vi "closePanel.vi"() -> ()   [LabVIEW 2015]
uses:
  GlobalPath.vi
  GlobalData.vi
  GlobalVi.vi
panel:
  out "Debug":string=" PANEL CLOSURE:"
  out "Stiffback XY Filename":string
  out "Micrometer Diff Filename":string
  out "PanelName":string
  in  "Done with gauge system?":bool
  in  "Done with micrometer?":bool
  in  "Open micrometer dry run":bool
  in  "Open Stiffback XY Program":bool
  in  "DONE ALL?":bool
  in  "ptfe 12":bool caption="Wait 24h for the glue to cure"
  in  "ptfe 11":bool caption="Remove the movement arch from over the table"
  in  "ptfe 8":bool caption="Position the weights on the stiffback"
  in  "ptfe 7":bool caption="Release the stiffback from the movement arch"
  in  "ptfe 6":bool caption="Lower the stiffback on the reference plates"
  in  "ptfe 5":bool caption="Move the stiffback over the reference plates"
  in  "ptfe 4":bool caption="Rotate the stiffback upside down"
  in  "ptfe 3":bool caption="Check cleanness of the 20 stiffback supports"
  in  "ptfe 2":bool caption="Move the stiffback away from the table"
  # "1. Panel Closure"
  # "2. Measurements"
  # "Micrometer measurement of the distance between the reference plates \nand the stiffback plates along the perimeter"
  # "Stiffback surface measurement (back side) with \ngauge system"
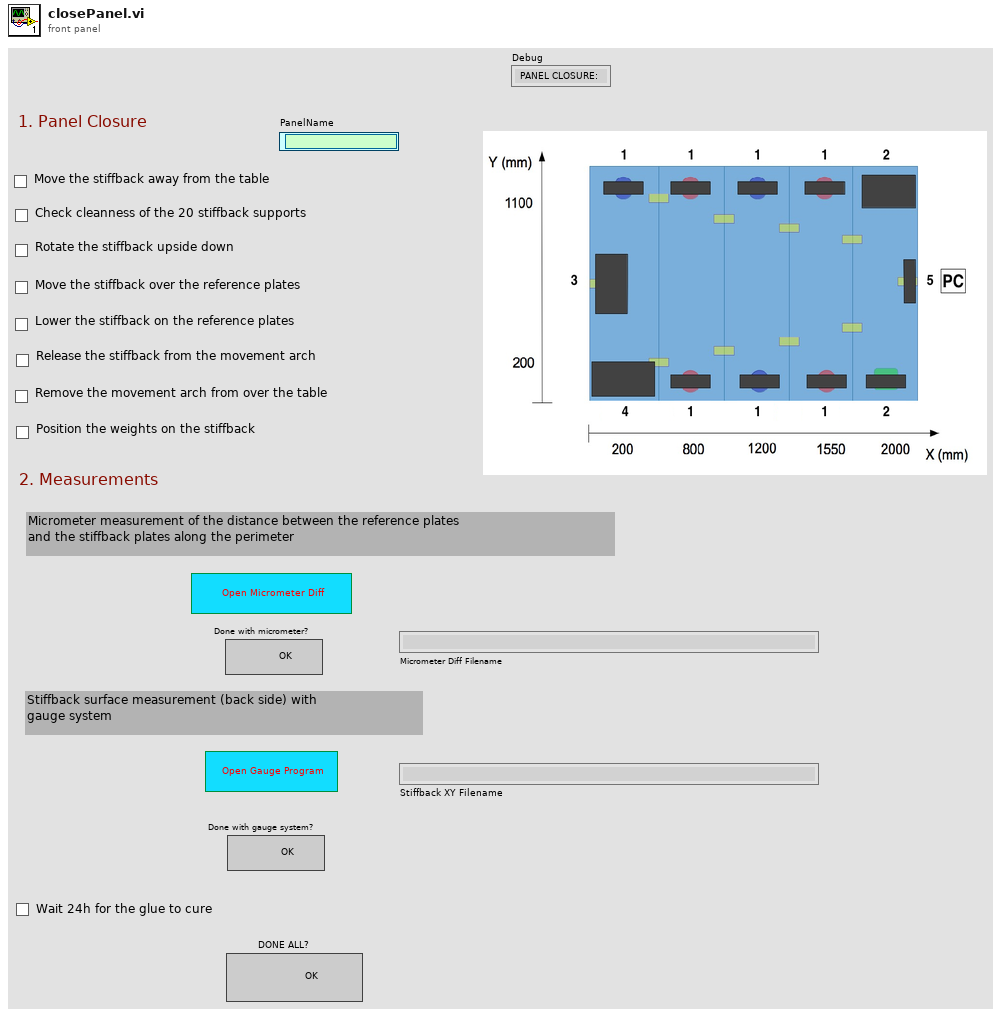
[diagram p1: front panel]
types:
  T1 = enum16{"open", "replace", "create", "open or create", "replace or create", "replace or create with confirmation"}
  T2 = enum32{"Bad", "Idle", "Run top level", "Running"}
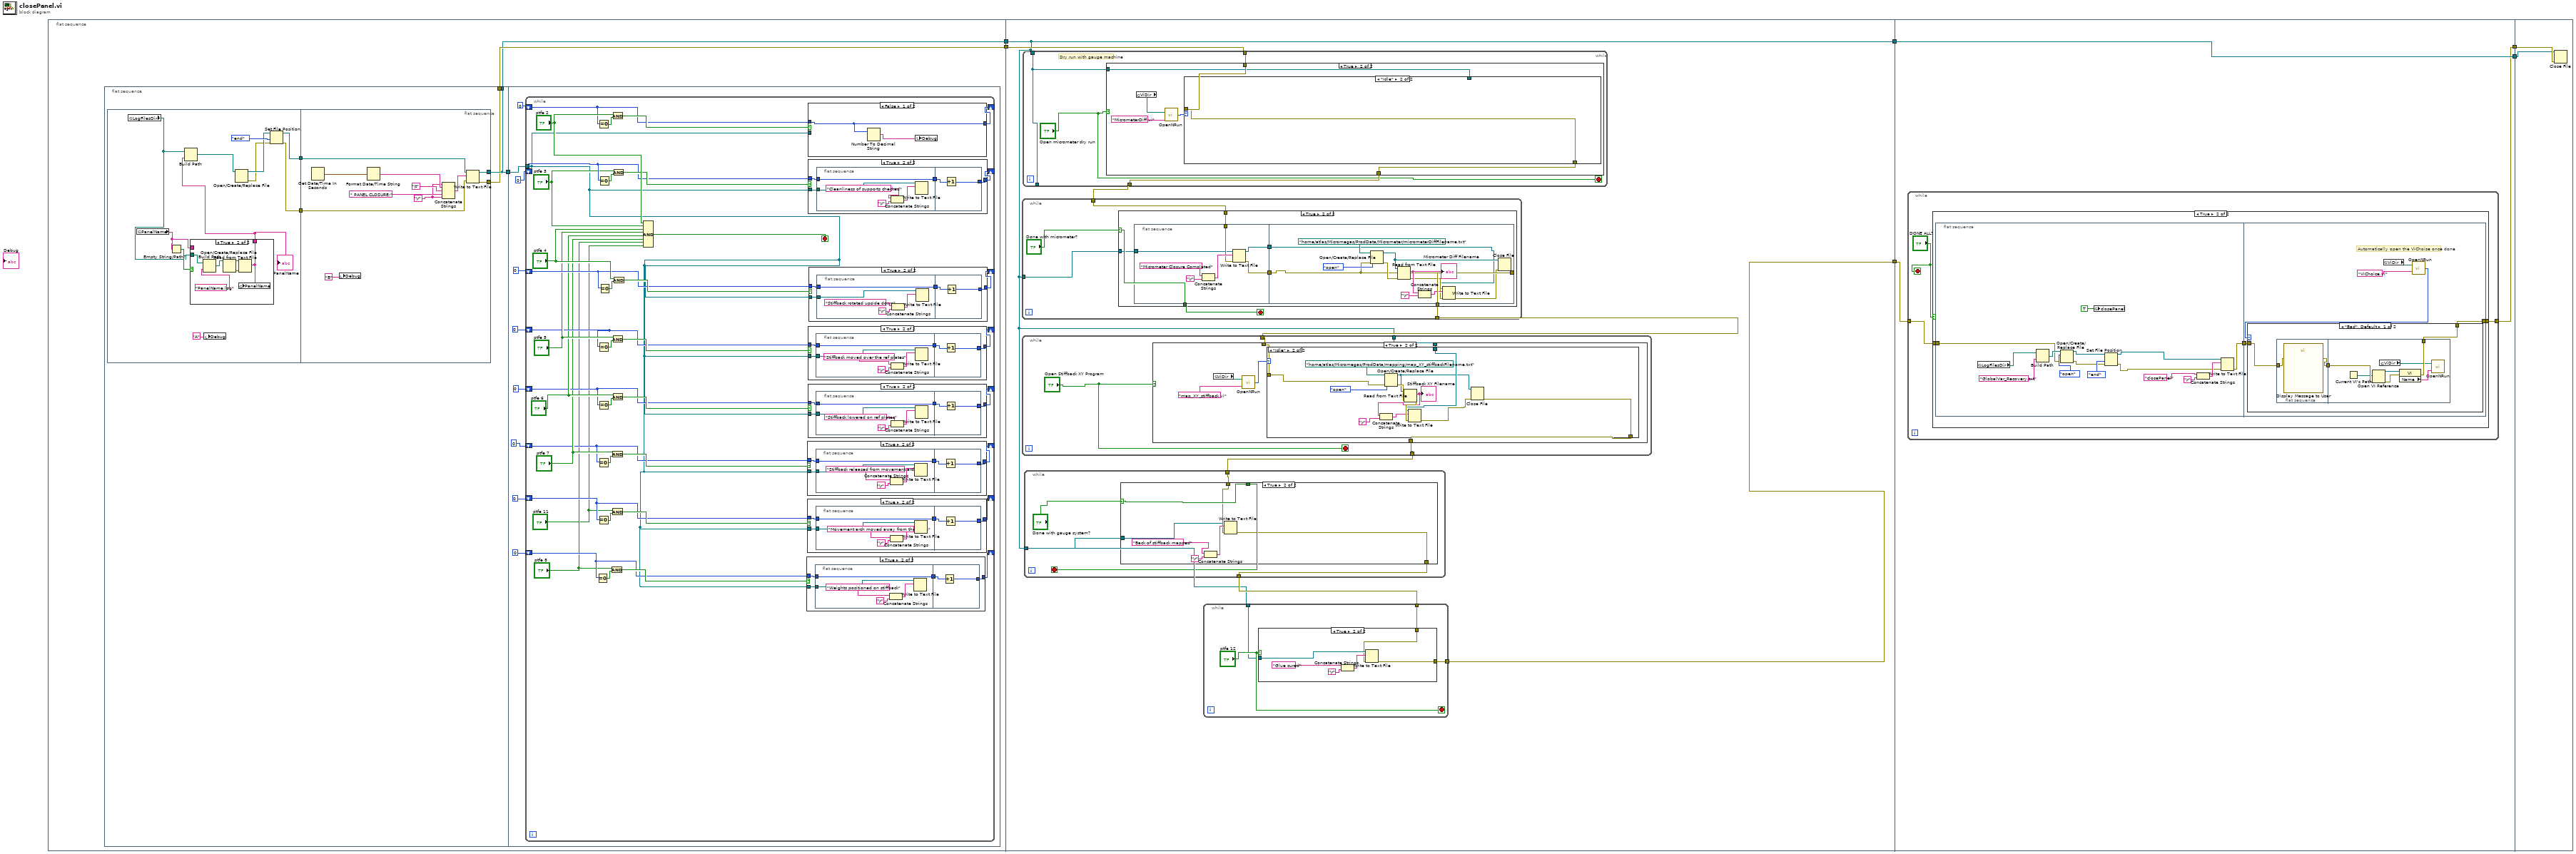
[diagram p0: block diagram]
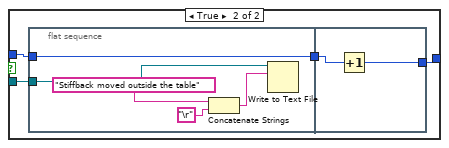
[diagram p10: hidden frame]
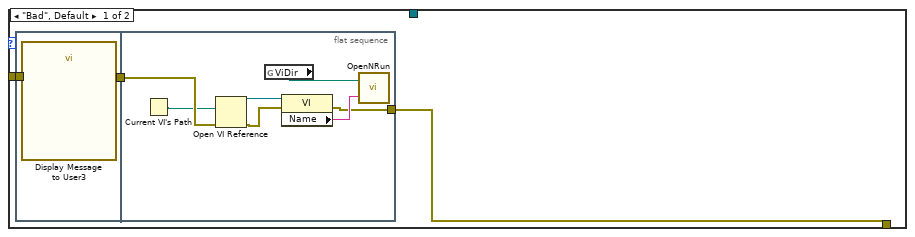
[diagram p14: hidden frame]
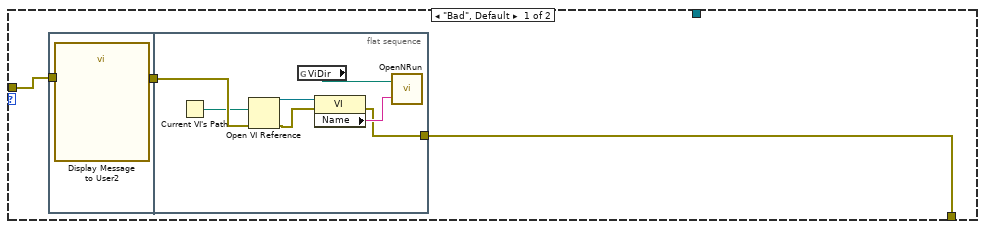
[diagram p16: hidden frame]
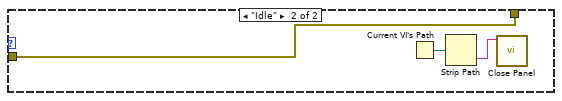
[diagram p19: hidden frame]
diagram:
  n1 = flat-sequence {
    tunnel: [w8] -> w4
    tunnel: [w7] -> w2
    tunnel: w4 -> [w197]
    tunnel: [w192] -> w3
    tunnel: w2 -> [w191]
    tunnel: [w191] -> w1
    tunnel: [w313] -> w6
    tunnel: w3 -> [w314]
    tunnel: w1 -> [w315]
    tunnel: [w315] -> w5
    tunnel: w6 -> [w359]
    tunnel: w5 -> [w358]
    frame #0 {
      n2 = flat-sequence {
        tunnel: [w12] -> w9
        tunnel: [w12] -> w7
        tunnel: [w11] -> w8
        tunnel: w9 -> [w51]
        frame #0 {
          n3 = flat-sequence {
            tunnel: [w22] -> w13
            tunnel: [w19] -> w10
            tunnel: w13 -> [w39]
            tunnel: [w38] -> w12
            tunnel: [w37] -> w11
            tunnel: w10 -> [w36]
            frame #0 {
              n4 = global read "GlobalPath.vi" "LogFilesDir"() -> (w15:path)
              n5 = global read "GlobalData.vi" "PanelName"() -> (w18:string)
              n6 = Empty String/Path?(string/path=w18) -> (empty?=w17:bool)
              n7 = case shown="True" w17 {
                tunnel: w15 -> [_ w31]
                tunnel: [w25 w26] -> w16
                tunnel: w18 -> [w25 _]
                frame False {
                }
                frame True {
                  n8 = Build Path(base path=w31, name or relative path="PanelName.log") -> (appended path=w30:path)
                  n9 = Open/Create/Replace File(file path (use dialog)=w30) -> (refnum out=w27:refnum<file>, error out=w28:errorcluster)  [unwired: 5 in, 1 out]
                  n10 = Read from Text File(file (use dialog)=w27, error in=w28) -> (text=w26:string)  [unwired: 2 in, 3 out]
                  n11 = global write "GlobalData.vi" "PanelName"(w26) -> ()
                }
              }
              "PanelName" <- w16
              n12 = Build Path(base path=w15, name or relative path=w16) -> (appended path=w24:path)
              n13 = local write "Debug"("A") -> ()
              n14 = Open/Create/Replace File(file path (use dialog)=w24) -> (refnum out=w21:refnum<file>, error out=w20:errorcluster)  [unwired: 5 in, 1 out]
              n15 = Set File Position(refnum=w21, from (0:start)=enum16{"start", "end", "current"}."end", error in=w20) -> (refnum out=w22:refnum<file>, error out=w19:errorcluster)  [unwired: 1 in]
            }
            frame #1 {
              w33 = "\r"
              n16 = Get Date/Time In Seconds() -> (seconds since 1Jan1904=w35:timestamp)
              n17 = local write "Debug"("B") -> ()
              n18 = Format Date/Time String(seconds (now)=w35) -> (date/time string=w41:string)  [unwired: 2 in]
              n19 = Concatenate Strings(w33, w41, "\t", " PANEL CLOSURE:", w33) -> (w40:string)
              n20 = Write to Text File(file (use dialog)=w39, text=w40, error in=w36) -> (refnum out=w38:refnum<file>, error out=w37:errorcluster)  [unwired: 1 in, 1 out]
            }
          }
        }
        frame #1 {
          n21 = while {
            tunnel: w51 -> [w53]
            shift-right: [w89] -> _
            shift-left: 0 -> [w52]
            shift-right: [w85] -> _
            shift-left: 0 -> [w86]
            shift-right: [w79] -> _
            shift-left: 0 -> [w80]
            shift-right: [w74] -> _
            shift-left: 0 -> [w75]
            shift-right: [w69] -> _
            shift-left: 0 -> [w70]
            shift-right: [w64] -> _
            shift-left: 0 -> [w65]
            shift-right: [w56] -> _
            shift-left: 0 -> [w59]
            shift-right: [w55] -> _
            shift-left: 0 -> [w58]
            stop <- w93 stop-if-true
            n22 = Equal To 0?(x=w58) -> (x = 0?=w61:bool)
            n23 = Equal To 0?(x=w65) -> (x = 0?=w68:bool)
            n24 = Equal To 0?(x=w59) -> (x = 0?=w63:bool)
            n25 = Equal To 0?(x=w52) -> (x = 0?=w92:bool)
            n26 = Equal To 0?(x=w75) -> (x = 0?=w78:bool)
            n27 = Equal To 0?(x=w70) -> (x = 0?=w73:bool)
            n28 = Equal To 0?(x=w86) -> (x = 0?=w88:bool)
            n29 = Equal To 0?(x=w80) -> (x = 0?=w83:bool)
            n30 = And(x="ptfe 8", y=w61) -> (x .and. y?=w60:bool)
            n31 = And(x="ptfe 7", y=w68) -> (x .and. y?=w67:bool)
            n32 = And(x="ptfe 11", y=w63) -> (x .and. y?=w62:bool)
            n33 = And(x="ptfe 2", y=w92) -> (x .and. y?=w91:bool)
            n34 = And(x="ptfe 5", y=w78) -> (x .and. y?=w77:bool)
            n35 = And(x="ptfe 6", y=w73) -> (x .and. y?=w72:bool)
            n36 = And(x="ptfe 3", y=w88) -> (x .and. y?=w87:bool)
            n37 = And(x="ptfe 4", y=w83) -> (x .and. y?=w82:bool)
            n38 = Compound Arithmetic op=AND("ptfe 2", "ptfe 3", "ptfe 4", "ptfe 5", "ptfe 6", "ptfe 7", "ptfe 8", "ptfe 11") -> (w93:bool)
            n39 = case shown="True" w60 {
              tunnel: w53 -> [_ w98]
              tunnel: w58 -> [w94 w96]
              tunnel: [w94 w95] -> w55
              frame False {
              }
              frame True {
                n40 = flat-sequence {
                  tunnel: w98 -> [w101]
                  tunnel: [w100] -> w97
                  tunnel: w96 -> [w100]
                  tunnel: w97 -> [w105]
                  tunnel: [w104] -> w95
                  frame #0 {
                    n41 = Concatenate Strings("Weights positioned on stiffback", "\r") -> (w103:string)
                    n42 = Write to Text File(file (use dialog)=w101, text=w103) -> ()  [unwired: 2 in, 3 out]
                  }
                  frame #1 {
                    n43 = Increment(x=w105) -> (x+1=w104:i32)
                  }
                }
              }
            }
            n44 = case shown="True" w67 {
              tunnel: w53 -> [_ w122]
              tunnel: w65 -> [w118 w120]
              tunnel: [w118 w119] -> w64
              frame False {
              }
              frame True {
                n45 = flat-sequence {
                  tunnel: w122 -> [w125]
                  tunnel: [w124] -> w121
                  tunnel: w120 -> [w124]
                  tunnel: w121 -> [w129]
                  tunnel: [w128] -> w119
                  frame #0 {
                    n46 = Concatenate Strings("Stiffback released from movement arch", "\r") -> (w127:string)
                    n47 = Write to Text File(file (use dialog)=w125, text=w127) -> ()  [unwired: 2 in, 3 out]
                  }
                  frame #1 {
                    n48 = Increment(x=w129) -> (x+1=w128:i32)
                  }
                }
              }
            }
            n49 = case shown="True" w62 {
              tunnel: w53 -> [_ w110]
              tunnel: w59 -> [w106 w108]
              tunnel: [w106 w107] -> w56
              frame False {
              }
              frame True {
                n50 = flat-sequence {
                  tunnel: w110 -> [w113]
                  tunnel: [w112] -> w109
                  tunnel: w108 -> [w112]
                  tunnel: w109 -> [w117]
                  tunnel: [w116] -> w107
                  frame #0 {
                    n51 = Concatenate Strings("Movement arch moved away from the table", "\r") -> (w115:string)
                    n52 = Write to Text File(file (use dialog)=w113, text=w115) -> ()  [unwired: 2 in, 3 out]
                  }
                  frame #1 {
                    n53 = Increment(x=w117) -> (x+1=w116:i32)
                  }
                }
              }
            }
            n54 = case shown="False" w91 {
              tunnel: w53 -> [_ w183]
              tunnel: w52 -> [w178 w181]
              tunnel: [w178 w180] -> w89
              frame False {
                n55 = Number To Decimal String(number=w178) -> (decimal integer string=w179:string)  [unwired: 1 in]
                n56 = local write "Debug"(w179) -> ()
              }
              frame True {
                n57 = flat-sequence {
                  tunnel: w183 -> [w186]
                  tunnel: [w185] -> w182
                  tunnel: w181 -> [w185]
                  tunnel: w182 -> [w190]
                  tunnel: [w189] -> w180
                  frame #0 {
                    n58 = Concatenate Strings("Stiffback moved outside the table", "\r") -> (w188:string)
                    n59 = Write to Text File(file (use dialog)=w186, text=w188) -> ()  [unwired: 2 in, 3 out]
                  }
                  frame #1 {
                    n60 = Increment(x=w190) -> (x+1=w189:i32)
                  }
                }
              }
            }
            n61 = case shown="True" w77 {
              tunnel: w53 -> [_ w146]
              tunnel: w75 -> [w142 w144]
              tunnel: [w142 w143] -> w74
              frame False {
              }
              frame True {
                n62 = flat-sequence {
                  tunnel: w146 -> [w149]
                  tunnel: [w148] -> w145
                  tunnel: w144 -> [w148]
                  tunnel: w145 -> [w153]
                  tunnel: [w152] -> w143
                  frame #0 {
                    n63 = Concatenate Strings("Stiffback moved over the ref plates", "\r") -> (w151:string)
                    n64 = Write to Text File(file (use dialog)=w149, text=w151) -> ()  [unwired: 2 in, 3 out]
                  }
                  frame #1 {
                    n65 = Increment(x=w153) -> (x+1=w152:i32)
                  }
                }
              }
            }
            n66 = case shown="True" w72 {
              tunnel: w53 -> [_ w134]
              tunnel: w70 -> [w130 w132]
              tunnel: [w130 w131] -> w69
              frame False {
              }
              frame True {
                n67 = flat-sequence {
                  tunnel: w134 -> [w137]
                  tunnel: [w136] -> w133
                  tunnel: w132 -> [w136]
                  tunnel: w133 -> [w141]
                  tunnel: [w140] -> w131
                  frame #0 {
                    n68 = Concatenate Strings("Stiffback lowered on ref plates", "\r") -> (w139:string)
                    n69 = Write to Text File(file (use dialog)=w137, text=w139) -> ()  [unwired: 2 in, 3 out]
                  }
                  frame #1 {
                    n70 = Increment(x=w141) -> (x+1=w140:i32)
                  }
                }
              }
            }
            n71 = case shown="True" w87 {
              tunnel: w53 -> [_ w170]
              tunnel: w86 -> [w166 w168]
              tunnel: [w166 w167] -> w85
              frame False {
              }
              frame True {
                n72 = flat-sequence {
                  tunnel: w170 -> [w173]
                  tunnel: [w172] -> w169
                  tunnel: w168 -> [w172]
                  tunnel: w169 -> [w177]
                  tunnel: [w176] -> w167
                  frame #0 {
                    n73 = Concatenate Strings("Cleanliness of supports checked", "\r") -> (w175:string)
                    n74 = Write to Text File(file (use dialog)=w173, text=w175) -> ()  [unwired: 2 in, 3 out]
                  }
                  frame #1 {
                    n75 = Increment(x=w177) -> (x+1=w176:i32)
                  }
                }
              }
            }
            n76 = case shown="True" w82 {
              tunnel: w53 -> [_ w158]
              tunnel: w80 -> [w154 w156]
              tunnel: [w154 w155] -> w79
              frame False {
              }
              frame True {
                n77 = flat-sequence {
                  tunnel: w158 -> [w161]
                  tunnel: [w160] -> w157
                  tunnel: w156 -> [w160]
                  tunnel: w157 -> [w165]
                  tunnel: [w164] -> w155
                  frame #0 {
                    n78 = Concatenate Strings("Stiffback rotated upside down", "\r") -> (w163:string)
                    n79 = Write to Text File(file (use dialog)=w161, text=w163) -> ()  [unwired: 2 in, 3 out]
                  }
                  frame #1 {
                    n80 = Increment(x=w165) -> (x+1=w164:i32)
                  }
                }
              }
            }
          }
        }
      }
    }
    frame #1 {
      n81 = while {
        tunnel: [w260] -> w196
        tunnel: w197 -> [w261]
        tunnel: [w258] -> _
        tunnel: w191 -> [w258]
        stop <- "Open micrometer dry run" stop-if-true
        # "Dry run with gauge machine"
        n82 = case shown="True" "Open micrometer dry run" {
          tunnel: w261 -> [w262 w268]
          tunnel: [w262 w263] -> w260
          tunnel: w258 -> [_ w264]
          frame False {
          }
          frame True {
            n83 = global read "GlobalPath.vi" "ViDir"() -> (w267:path)
            n84 = call "OpenNRun.vi"("VI name"="MicrometerDiff.vi", "ViDirPath"=w267) -> ("Execution:State"=w266:T2)
            n85 = case shown="\"Idle\"" w266 {
              tunnel: w268 -> [w270 w281]
              tunnel: w264 -> [_ _]
              tunnel: [w269 w281] -> w263
              frame "Bad", Default {
                n86 = flat-sequence {
                  tunnel: [w273] -> w271
                  tunnel: w270 -> [w272]
                  tunnel: w271 -> [w276]
                  tunnel: [w274] -> w269
                  frame #0 {
                    n87 = call "Display Message to User2"("error in (no error)"=w272) -> ("error out"=w273:errorcluster)  [unwired: 9 in, 1 out]
                  }
                  frame #1 {
                    n88 = Current VI's Path() -> (path=w275:path)
                    n89 = Open VI Reference(vi path=w275, error in (no error)=w276) -> (vi reference=w280:refnum<vi>, error out=w279:errorcluster)  [unwired: 4 in]
                    n90 = global read "GlobalPath.vi" "ViDir"() -> (w278:path)
                    n91 = property class="VI"(reference=w280, error in=w279) -> (error out=w274:errorcluster, "Name"=w277:string)  [unwired: 1 out]
                    n92 = call "OpenNRun.vi"("VI name"=w277, "ViDirPath"=w278) -> ()  [unwired: 1 out]
                  }
                }
              }
              frame "Idle" {
              }
            }
          }
        }
      }
      n93 = while {
        tunnel: w196 -> [w285]
        tunnel: w191 -> [w284]
        tunnel: [w282] -> w195
        stop <- w286 stop-if-true
        n94 = case shown="True" "Done with micrometer?" {
          selector: "Done with micrometer?" -> [w288 w294]
          tunnel: [w288 w294] -> w286
          tunnel: w285 -> [w287 w293]
          tunnel: [w287 w291] -> w282
          tunnel: w284 -> [_ w292]
          frame False {
          }
          frame True {
            n95 = flat-sequence {
              tunnel: w293 -> [w298]
              tunnel: w292 -> [w297]
              tunnel: [w295] -> w290
              tunnel: [w296] -> w289
              tunnel: [w302] -> w291
              tunnel: w290 -> [w302]
              tunnel: w289 -> [w303]
              frame #0 {
                n96 = Concatenate Strings("Micrometer Closure Completed", "\r") -> (w301:string)
                n97 = Write to Text File(file (use dialog)=w297, text=w301, error in=w298) -> (refnum out=w296:refnum<file>, error out=w295:errorcluster)  [unwired: 1 in, 1 out]
              }
              frame #1 {
                n98 = Open/Create/Replace File(file path (use dialog)=path "/home/atlas/Micromegas/ProdData/Micrometer/micrometerDiffFilename.txt", error in=w302, operation (0:open)=T1."open") -> (refnum out=w311:refnum<file>, error out=w306:errorcluster)  [unwired: 3 in, 1 out]
                n99 = Read from Text File(file (use dialog)=w311, error in=w306) -> (text=w310:string, error out=w307:errorcluster)  [unwired: 2 in, 2 out]
                "Micrometer Diff Filename" <- w310
                n100 = Concatenate Strings(w310, "\r") -> (w308:string)
                n101 = Write to Text File(file (use dialog)=w303, text=w308, error in=w307) -> (error out=w312:errorcluster)  [unwired: 1 in, 2 out]
                n102 = Close File(refnum=w311, error in=w312) -> ()  [unwired: 2 out]
              }
            }
          }
        }
      }
      n103 = while {
        tunnel: [w226] -> w194
        tunnel: w195 -> [w225]
        tunnel: w191 -> [w223]
        stop <- "Open Stiffback XY Program" stop-if-true
        n104 = case shown="True" "Open Stiffback XY Program" {
          tunnel: [w227 w228] -> w226
          tunnel: w225 -> [w227 w231]
          tunnel: w223 -> [_ w229]
          frame False {
          }
          frame True {
            n105 = global read "GlobalPath.vi" "ViDir"() -> (w233:path)
            n106 = call "OpenNRun.vi"("VI name"="map_XY_stiffback.vi", "ViDirPath"=w233) -> ("Execution:State"=w232:T2)
            n107 = case shown="\"Idle\"" w232 {
              tunnel: w231 -> [w235 w250]
              tunnel: w229 -> [_ w249]
              tunnel: [w234 w247] -> w228
              frame "Bad", Default {
                n108 = flat-sequence {
                  tunnel: [w237] -> w236
                  tunnel: w235 -> [w238]
                  tunnel: w236 -> [w241]
                  tunnel: [w239] -> w234
                  frame #0 {
                    n109 = call "Display Message to User3"("error in (no error)"=w238) -> ("error out"=w237:errorcluster)  [unwired: 9 in, 1 out]
                  }
                  frame #1 {
                    n110 = Current VI's Path() -> (path=w240:path)
                    n111 = Open VI Reference(vi path=w240, error in (no error)=w241) -> (vi reference=w245:refnum<vi>, error out=w244:errorcluster)  [unwired: 4 in]
                    n112 = global read "GlobalPath.vi" "ViDir"() -> (w243:path)
                    n113 = property class="VI"(reference=w245, error in=w244) -> (error out=w239:errorcluster, "Name"=w242:string)  [unwired: 1 out]
                    n114 = call "OpenNRun.vi"("VI name"=w242, "ViDirPath"=w243) -> ()  [unwired: 1 out]
                  }
                }
              }
              frame "Idle" {
                n115 = Open/Create/Replace File(file path (use dialog)=path "/home/atlas/Micromegas/ProdData/mapping/map_XY_stiffbackFilename.txt", error in=w250, operation (0:open)=T1."open") -> (refnum out=w246:refnum<file>, error out=w255:errorcluster)  [unwired: 3 in, 1 out]
                n116 = Read from Text File(file (use dialog)=w246, error in=w255) -> (text=w251:string, error out=w254:errorcluster)  [unwired: 2 in, 2 out]
                "Stiffback XY Filename" <- w251
                n117 = Concatenate Strings(w251, "\r") -> (w253:string)
                n118 = Write to Text File(file (use dialog)=w249, text=w253, error in=w254) -> (error out=w248:errorcluster)  [unwired: 1 in, 2 out]
                n119 = Close File(refnum=w246, error in=w248) -> (error out=w247:errorcluster)  [unwired: 1 out]
              }
            }
          }
        }
      }
      n120 = while {
        tunnel: w194 -> [w212]
        tunnel: w191 -> [w211]
        tunnel: [w209] -> w193
        stop <- w213 stop-if-true
        n121 = case shown="True" "Done with gauge system?" {
          selector: "Done with gauge system?" -> [w215 w220]
          tunnel: [w215 w220] -> w213
          tunnel: w212 -> [w214 w219]
          tunnel: w211 -> [_ w218]
          tunnel: [w214 w216] -> w209
          frame False {
          }
          frame True {
            n122 = Concatenate Strings("Back of stiffback mapped", "\r") -> (w222:string)
            n123 = Write to Text File(file (use dialog)=w218, text=w222, error in=w219) -> (error out=w216:errorcluster)  [unwired: 1 in, 2 out]
          }
        }
      }
      n124 = while {
        tunnel: w191 -> [w200]
        tunnel: w193 -> [w199]
        tunnel: [w198] -> w192
        stop <- "ptfe 12" stop-if-true
        n125 = case shown="True" "ptfe 12" {
          tunnel: w200 -> [_ w208]
          tunnel: w199 -> [w202 w204]
          tunnel: [w202 w203] -> w198
          frame False {
          }
          frame True {
            n126 = Concatenate Strings("Glue cured", "\r") -> (w207:string)
            n127 = Write to Text File(file (use dialog)=w208, text=w207, error in=w204) -> (error out=w203:errorcluster)  [unwired: 1 in, 2 out]
          }
        }
      }
    }
    frame #2 {
      n128 = while {
        tunnel: w314 -> [w318]
        tunnel: [w317] -> w313
        stop <- "DONE ALL?" stop-if-true
        n129 = case shown="True" "DONE ALL?" {
          tunnel: [w319 w322] -> w317
          tunnel: w318 -> [w319 w320]
          frame False {
          }
          frame True {
            n130 = flat-sequence {
              tunnel: [w326] -> w321
              tunnel: w320 -> [w325]
              tunnel: [w339] -> w322
              tunnel: w321 -> [w338]
              frame #0 {
                n131 = global read "GlobalPath.vi" "LogFilesDir"() -> (w323:path)
                n132 = Build Path(base path=w323, name or relative path="GlobalVar_Recovery.txt") -> (appended path=w335:path)
                n133 = Open/Create/Replace File(file path (use dialog)=w335, error in=w325, operation (0:open)=T1."open") -> (refnum out=w331:refnum<file>, error out=w332:errorcluster)  [unwired: 3 in, 1 out]
                n134 = global write "GlobalVi.vi" "closePanel"(TRUE) -> ()
                n135 = Set File Position(refnum=w331, from (0:start)=enum16{"start", "end", "current"}."end", error in=w332) -> (refnum out=w328:refnum<file>, error out=w327:errorcluster)  [unwired: 1 in]
                n136 = Concatenate Strings("closePanel", "\r") -> (w330:string)
                n137 = Write to Text File(file (use dialog)=w328, text=w330, error in=w327) -> (error out=w326:errorcluster)  [unwired: 1 in, 2 out]
              }
              frame #1 {
                # "Automatically open the ViChoise once done"
                n138 = global read "GlobalPath.vi" "ViDir"() -> (w342:path)
                n139 = call "OpenNRun.vi"("VI name"="ViChoice.vi", "ViDirPath"=w342) -> ("Execution:State"=w341:T2)
                n140 = case shown="\"Bad\", Default" w341 {
                  tunnel: [w343 w355] -> w339
                  tunnel: w338 -> [w344 w355]
                  frame "Bad", Default {
                    n141 = flat-sequence {
                      tunnel: w344 -> [w347]
                      tunnel: [w346] -> w345
                      tunnel: [w351] -> w343
                      tunnel: w345 -> [w350]
                      frame #0 {
                        n142 = call "Display Message to User"("error in (no error)"=w347) -> ("error out"=w346:errorcluster)  [unwired: 9 in, 1 out]
                      }
                      frame #1 {
                        n143 = Current VI's Path() -> (path=w348:path)
                        n144 = Open VI Reference(vi path=w348, error in (no error)=w350) -> (vi reference=w354:refnum<vi>, error out=w353:errorcluster)  [unwired: 4 in]
                        n145 = global read "GlobalPath.vi" "ViDir"() -> (w349:path)
                        n146 = property class="VI"(reference=w354, error in=w353) -> (error out=w351:errorcluster, "Name"=w352:string)  [unwired: 1 out]
                        n147 = call "OpenNRun.vi"("VI name"=w352, "ViDirPath"=w349) -> ()  [unwired: 1 out]
                      }
                    }
                  }
                  frame "Idle" {
                    n148 = Current VI's Path() -> (path=w356:path)
                    n149 = Strip Path(path=w356) -> (name=w357:string)  [unwired: 1 out]
                    n150 = call <vilib>:"Close Panel.vi"("VI name"=w357) -> ()  [unwired: 10 in, 1 out]
                  }
                }
              }
            }
          }
        }
      }
    }
    frame #3 {
      n151 = Close File(refnum=w358, error in=w359) -> ()  [unwired: 2 out]
    }
  }
